vi "Import as Child.vi"(8 "error in":errorcluster, 9 "name":string, 10 "path":path, 11 "parent ref in":T1 format="%.0x") -> (0 "error out":errorcluster, 2 "new item ref":T1 format="%.0x", 3 "parent ref out":T1 format="%.0x")   [LabVIEW 2027, in "Custom Device Serialization.lvlib"]
uses:
  Custom Device Serialization.lvlib
  <vilib>/NI VeriStand/Custom Device API/Custom Device Item Ref.ctl
  <vilib>/NI VeriStand/Custom Device API/Custom Device API.lvlib
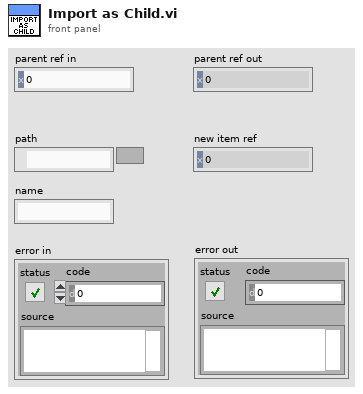
[diagram p1: front panel]
types:
  T1 = typedef "Custom Device API.lvlib/Custom Device Item Ref.ctl" = u64
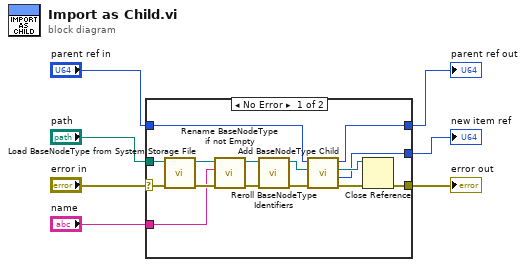
[diagram p0: block diagram]
diagram:
  n1 = case shown="No Error" "error in" {
    selector: "error in" -> [w21 w24]
    tunnel: "path" -> [w22 _]
    tunnel: [w18 w24] -> w5
    tunnel: "parent ref in" -> [w17 w23]
    tunnel: [w16 _] -> w4
    tunnel: [w15 w23] -> w2
    tunnel: "name" -> [w8 _]
    frame No Error {
      n2 = call "Load BaseNodeType from System Storage File.vi"("error in (no error)"=w21, "path"=w22) -> ("error out"=w14:errorcluster, "NationalInstruments.VeriStand.SystemStorage.BaseNodeType"=w10:refnum<k39>)  [unwired: 8 in]
      n3 = call "Rename BaseNodeType if not Empty.vi"("error in"=w14, "name"=w8, "NationalInstruments.VeriStand.SystemStorage.BaseNodeType"=w10) -> ("error out"=w11:errorcluster, "NationalInstruments.VeriStand.SystemStorage.BaseNodeType"=w9:refnum<k39>)  [unwired: 7 in]
      n4 = call "Reroll BaseNodeType Identifiers.vi"("error in"=w11, "NationalInstruments.VeriStand.SystemStorage.BaseNodeType"=w9) -> ("error out"=w12:errorcluster, "NationalInstruments.VeriStand.SystemStorage.BaseNodeType"=w13:refnum<k39>)  [unwired: 8 in]
      n5 = call "Add BaseNodeType Child.vi"("error in"=w12, "NationalInstruments.VeriStand.SystemStorage.BaseNodeType"=w13, "parent ref in"=w17) -> ("error out"=w19:errorcluster, "child ref"=w16:T1, "NationalInstruments.VeriStand.SystemStorage.BaseNodeType"=w20:refnum<k39>, "parent ref out"=w15:T1)  [unwired: 5 in]
      n6 = Close Reference(reference=w20, error in (no error)=w19) -> (error out=w18:errorcluster)
    }
    frame Error {
    }
  }
  "error out" <- w5
  "new item ref" <- w4
  "parent ref out" <- w2
